vi "Maxi Gauge-RW Interface.vi"(7 "W/R":bool, 8 "Fehler (Eingang)":errorcluster, 9 "Interface Set":u8(ring) items=["R232", "RS422", "RS422 I", "RS485 I"], 10 "Node address":i8=-1 min=-1 max=31 step=1, 11 "VISA-Ressource in":refnum<visa-resource-name>) -> (0 "Fehler (Ausgang)":errorcluster, 1 "Interface Get":u8(ring) items=["R232", "RS422", "RS422 I", "RS485 I"], 3 "VISA-Ressource out":refnum<visa-resource-name>)   [LabVIEW 2013, in "Maxi Gauge.lvlib"]
uses:
  <instrlib>/Maxi Gauge/Maxi Gauge.lvlib
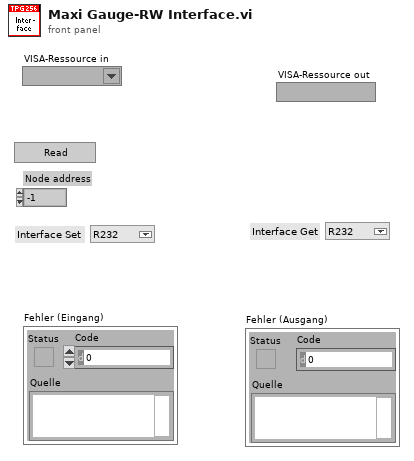
[diagram p1: front panel]
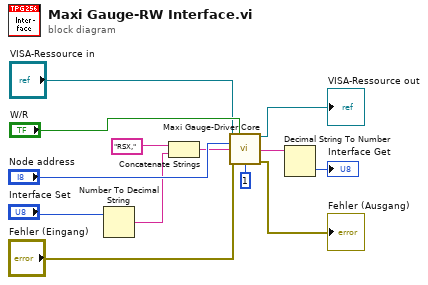
[diagram p0: block diagram]
diagram:
  n1 = Number To Decimal String(number="Interface Set") -> (decimal integer string=w8:string)  [unwired: 1 in]
  n2 = Concatenate Strings("RSX," ("Command"), w8) -> (w5:string)
  n3 = call <instrlib>:"Maxi Gauge-Driver Core.vi"("VISA-Ressource in"="VISA-Ressource in", "Write/Read"="W/R", "Node address"="Node address", "Command"=w5, "Fehler (Eingang)"="Fehler (Eingang)", "Retry (3)"=1) -> ("VISA-Ressource out"=→"VISA-Ressource out":refnum<visa-resource-name>, "String Out"=w7:string, "Fehler (Ausgang)"=→"Fehler (Ausgang)":errorcluster)  [unwired: 7 in]
  n4 = Decimal String To Number(string=w7) -> (number=→"Interface Get":i32)  [unwired: 2 in, 1 out]
